vi "Pickup Command.vi"(6 "Synchronization":enum16{"Start", "Wait"}(ring), 7 "Description":string, 8 "Command Info In":T3) -> (0 "Command Info Out":T3)   [LabVIEW 2018]
doc: "This template has a parameter to control whether it waits for the command to complete or not. This is useful for operations that have a timed duration or a sensor-based duration. \n\nBe sure to right-click and select New from Template and save with a new command name."
uses:
  Implementation/Subsystem Sequencer Operations.ctl
  Implementation/Subsystem Sequencer Setpoints.ctl
  <vilib>/Rock Robotics/WPI/Framework/Completion Status.ctl
  <vilib>/Rock Robotics/WPI/Framework/Completion Notifier.ctl
  <vilib>/Rock Robotics/WPI/Framework/Command Status Info.ctl
  Implementation/All Commands.ctl
  Implementation/Sequencer Type.ctl
panel:
  in  "Sequence":T1[](array[typedef])=[{"Cmd"=enum."Elevator - Elevator Set Position Start", "Value"=0.0}, {"Cmd"=enum."Arm - Arm to Pickup Position", "Value"=0.0}, {"Cmd"=enum."Gripper - Gripper Open", "Value"=0.0}, {"Cmd"=enum."Gripper - Gripper Intake", "Value"=0.0}, {"Cmd"=enum."Gripper - Wait on Sensor", "Value"=0.0}, {"Cmd"=enum."Gripper - Gripper Close", "Value"=0.0}, {"Cmd"=enum."Gripper - Gripper Stop", "Value"=0.0}, {"Cmd"=enum."Wait ms", "Value"=100.0}, {"Cmd"=enum."Arm - Arm to Shoot Position", "Value"=0.0}]
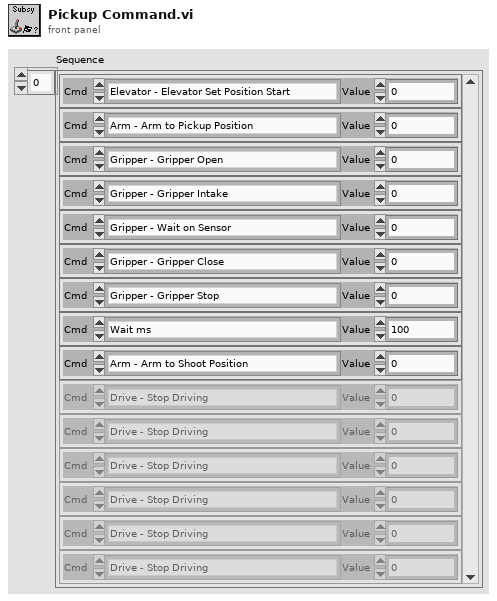
[diagram p1: front panel]
types:
  T1 = typedef "Sequencer Type.ctl" = cluster{"Cmd":T2, "Value":dbl}
  T2 = typedef "All Commands.ctl" = enum16{"Wait ms", "Drive - Stop Driving", "Drive - Set Shifter", "Drive - Drive Distance Straight", "Elevator - Elevator Stop", "Elevator - Elevator Set Position Wait", "Elevator - Elevator Set Position Start", "Arm - Arm to Shoot Position", "Arm - Arm to Pickup Position", "Arm - Arm Set Position", "Gripper - Gripper Stop", "Gripper - Gripper Shoot", "Gripper - Gripper Open", "Gripper - Gripper Intake", "Gripper - Gripper Close", "Gripper - Wait on Sensor"}
  T3 = typedef "Command Status Info.ctl" = cluster{"Name":string, "Status":T4, "notifier out":T5}
  T4 = typedef "Completion Status.ctl" = enum16{"Successful", "Aborted", "Incomplete"}
  T5 = typedef "Completion Notifier.ctl" = refnum<notifier>
  T6 = typedef "Subsystem Sequencer Setpoints.ctl" = cluster{"Operation":T7, "Setpoint":dbl, "Duration":dbl}
  T7 = typedef "Subsystem Sequencer Operations.ctl" = enum16{"Reserve", "Read Current", "Run Sequence"}
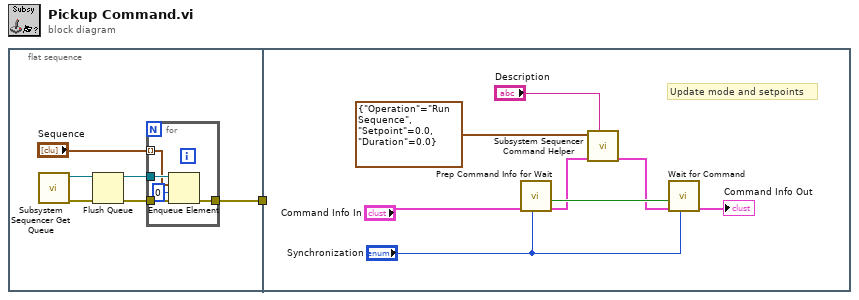
[diagram p0: block diagram]
diagram:
  n1 = flat-sequence {
    tunnel: [w2] -> w1
    tunnel: w1 -> [_]
    frame #0 {
      n2 = call "Subsystem Sequencer Get Queue.vi"() -> ("error out"=w7:errorcluster, "queue out"=w4:refnum<queue>)  [unwired: 10 in]
      n3 = Flush Queue(queue=w4, error in (no error)=w7) -> (queue out=w3:refnum<queue>, error out=w5:errorcluster)  [unwired: 1 out]
      n4 = for {
        tunnel: w3 -> [w12]
        tunnel: w5 -> [w11]
        tunnel: "Sequence" -> [w10] mode=indexing
        tunnel: [w8] -> w2
        n5 = Enqueue Element(queue=w12, element=w10, timeout in ms (-1)=0, error in (no error)=w11) -> (error out=w8:errorcluster)  [unwired: 2 out]
      }
    }
    frame #1 {
      # "Update mode and setpoints"
      n6 = call <vilib>:"Prep Command Info for Wait.vi"("Synchronication"="Synchronization", "Command Info"="Command Info In") -> ("Command Info"=w18:T3, "Allocated"=w19:bool)  [unwired: 8 in]
      n7 = call "Subsystem Sequencer Command Helper.vi"("Description"="Description", "Command Info In"=w18, "SubSystem Data"=T6 {"Operation"=enum."Run Sequence", "Setpoint"=0.0, "Duration"=0.0}) -> ("Command Info Out"=w15:T3)  [unwired: 6 in, 2 out]
      n8 = call <vilib>:"Wait for Command.vi"("Synchronication"="Synchronization", "Command Info in"=w15, "Allocated"=w19) -> ("Command Info out"=→"Command Info Out":T3)  [unwired: 8 in]
    }
  }
